vi "GetStrideElementCnt.vi"(3 "ndims":i32, 4 "shape":u64[](array[numeric]), 5 "CurrentIndex":u64[](array[numeric])) -> (0 "shape[i-1]":u64, 1 "shape[i-2]":u64, 2 "strideElementCnt":u64)   [LabVIEW 2016]
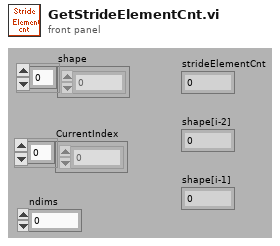
[diagram p1: front panel]
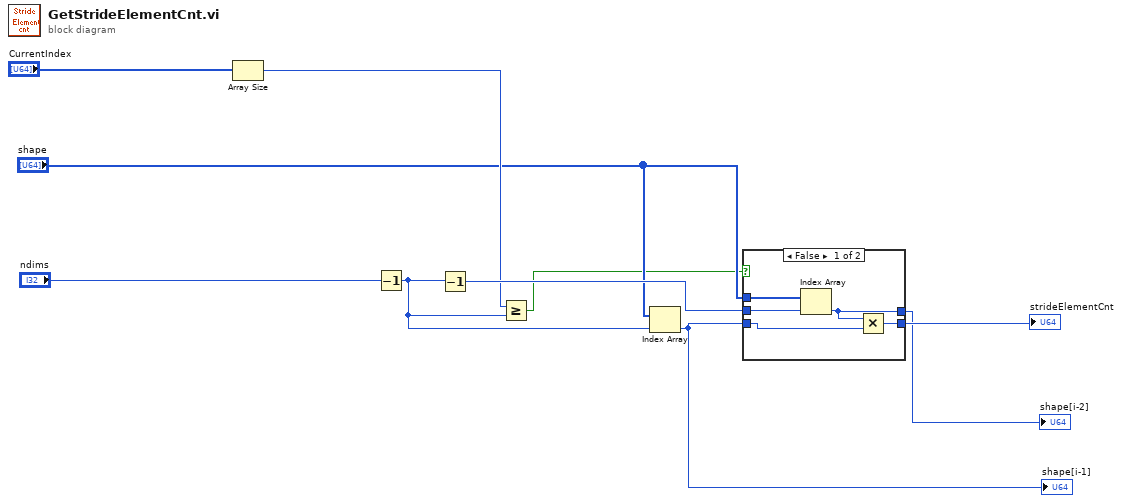
[diagram p0: block diagram]
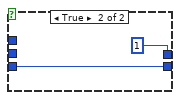
[diagram p2: hidden frame]
diagram:
  n1 = Array Size(array="CurrentIndex") -> (size(s)=w5:i32)
  n2 = Decrement(x="ndims") -> (x-1=w3:i32)
  n3 = Decrement(x=w3) -> (x-1=w10:i32)
  n4 = Greater Or Equal?(x=w5, y=w3) -> (x >= y?=w1:bool)
  n5 = Index Array(array="shape", index=w3) -> (element=w7:u64)
  "shape[i-1]" <- w7
  n6 = case shown="False" w1 {
    tunnel: "shape" -> [w15 _]
    tunnel: w10 -> [w14 _]
    tunnel: w7 -> [w13 w17]
    tunnel: [w12 w17] -> w9
    tunnel: [w11 u64 1 ("数值")] -> w8
    frame False {
      n7 = Index Array(array=w15, index=w14) -> (element=w11:u64)
      n8 = Multiply(x=w11, y=w13) -> (x*y=w12:u64)
    }
    frame True {
    }
  }
  "strideElementCnt" <- w9
  "shape[i-2]" <- w8
